vi "Configure PRBS Waveform.vi"(4 "Offset (0.00 V)":dbl min=-10.0 max=10.0, 5 "Amplitude (4 Vpp)":dbl=4.0, 6 "Edge Time (10 ns)":dbl=1e-08, 7 "Length (3)":u16=3, 8 "error in (no error)":errorcluster, 9 "Bit Rate (1000 bits/second)":dbl=1000.0, 10 "Channel (1: 1)":u16(ring)=1 items=["Channel 1"=1, "Channel 2"=2], 11 "VISA resource name":refnum<visa-resource-name>) -> (0 "error out":errorcluster, 3 "VISA resource name out":refnum<visa-resource-name>)   [LabVIEW 2015, in "SDG X Series.lvlib"]
doc: "Configures PRBS waveform and parameters.\n\nNote:\nThis VI only supports SDG6000X series."
uses:
  <instrlib>/SDG X Series/SDG X Series.lvlib
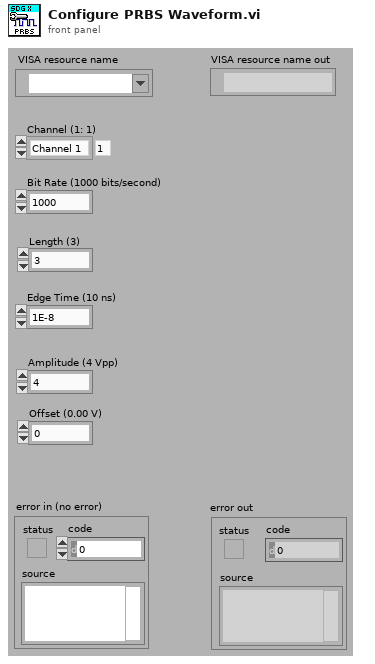
[diagram p1: front panel]
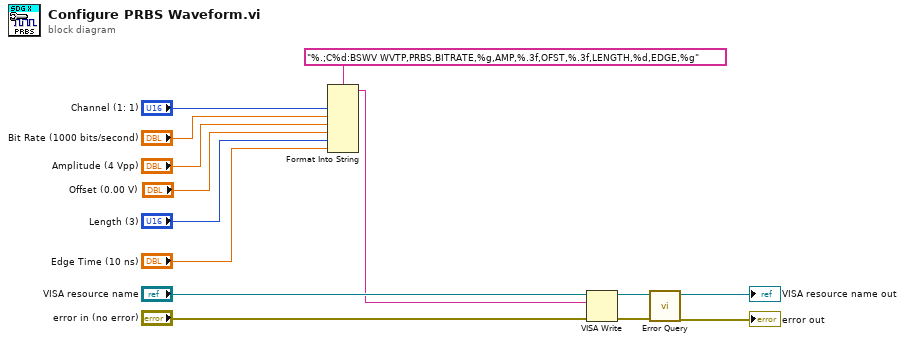
[diagram p0: block diagram]
diagram:
  n1 = Format Into String(format string="%.;C%d:BSWV WVTP,PRBS,BITRATE,%g,AMP,%.3f,OFST,%.3f,LENGTH,%d,EDGE,%g", "Channel (1: 1)", "Bit Rate (1000 bits/second)", "Amplitude (4 Vpp)", "Offset (0.00 V)", "Length (3)", "Edge Time (10 ns)") -> (resulting string=w1:string)  [unwired: 2 in, 1 out]
  n2 = VISA Write(VISA resource name="VISA resource name", write buffer=w1, error in (no error)="error in (no error)") -> (VISA resource name out=w12:refnum<visa-resource-name>, error out=w11:errorcluster)  [unwired: 1 out]
  n3 = call <instrlib>:"Error Query.vi"("error in (no error)"=w11, "VISA resource name"=w12) -> ("error out"=→"error out":errorcluster, "VISA resource name out"=→"VISA resource name out":refnum<visa-resource-name>)  [unwired: 6 in, 2 out]
